vi "Set_Device_NameIP.vi"(5 "Unit ID":u8, 6 "Timeout(ms)":i32, 7 "Device Name":string, 8 "error in (no error)":errorcluster, 9 "Port":u16, 10 "Device Address":string, 11 "Device in":refnum<class "DAQ_Device.lvclass">) -> (0 "error out":errorcluster, 3 "Device out":refnum<class "DAQ_Device.lvclass">)   [LabVIEW 2023, in "DAQ_Device.lvclass"]
uses:
  DAQ_Device.lvclass
  DAQ_Device.lvclass/DAQ_Device.ctl
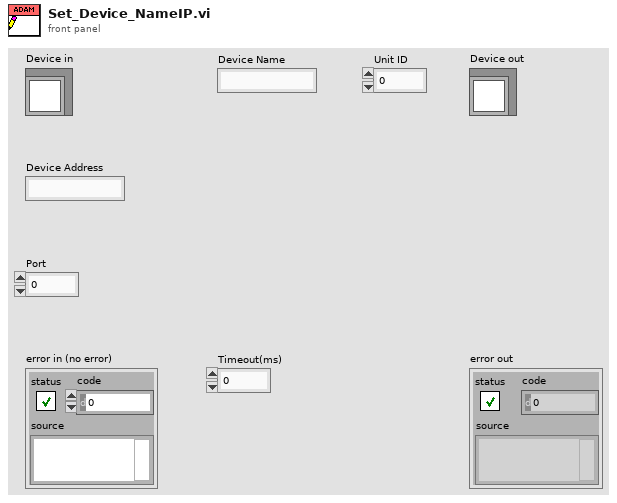
[diagram p1: front panel]
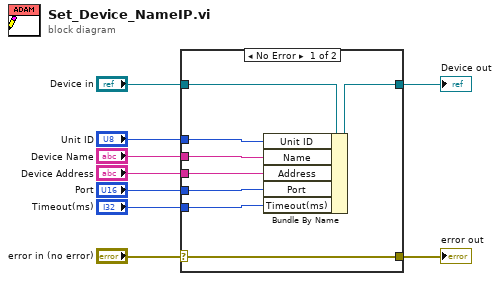
[diagram p0: block diagram]
diagram:
  n1 = case shown="No Error" "error in (no error)" {
    selector: "error in (no error)" -> [w17 w18]
    tunnel: [w17 w18] -> w8
    tunnel: [w15 w19] -> w6
    tunnel: "Device in" -> [w16 w19]
    tunnel: "Device Address" -> [w14 _]
    tunnel: "Port" -> [w13 _]
    tunnel: "Timeout(ms)" -> [w12 _]
    tunnel: "Device Name" -> [w11 _]
    tunnel: "Unit ID" -> [w10 _]
    frame No Error {
      n2 = Bundle By Name(cluster=w16, "Unit ID"=w10, "Name"=w11, "Address"=w14, "Port"=w13, "Timeout(ms)"=w12) -> (w15:refnum<class "DAQ_Device.lvclass">)
    }
    frame Error {
    }
  }
  "error out" <- w8
  "Device out" <- w6
